vi "Collector.vi"(11 "MechanismMetrics in":T1) -> (3 "MechanismMetrics out":T1)   [LabVIEW 2014]
uses:
  <vilib>/Rock Robotics/WPI/Solenoid/WPI_SolenoidValue.ctl
  Lifter States.ctl
  <vilib>/Rock Robotics/WPI/Solenoid/WPI_SolenoidSetEnum.vi
  MechanismMetrics.ctl
  Auto Lifter States.ctl
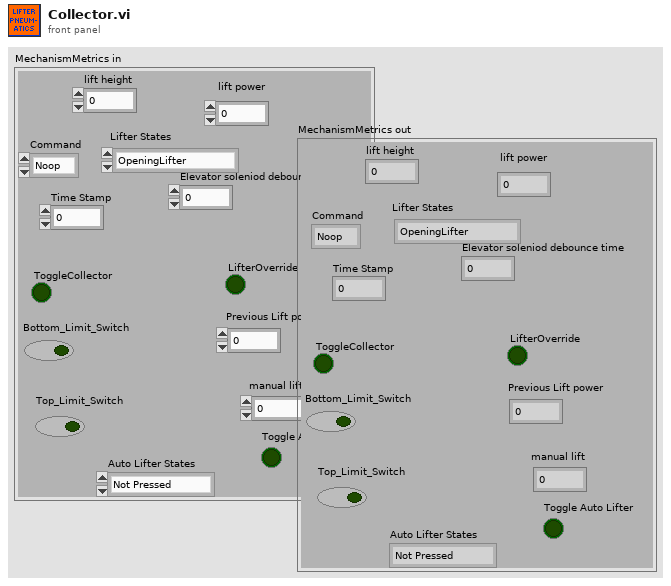
[diagram p1: front panel]
types:
  T1 = typedef "MechanismMetrics.ctl" = cluster{"lift height":dbl, "Command":enum16{"Noop", "Flagged"}, "Time Stamp":u32, "ToggleCollector":bool, "Bottom_Limit_Switch ":bool, "Top_Limit_Switch":bool, "lift power":dbl, "Elevator soleniod debounce time   ":dbl, "LifterOverride":bool, "Previous Lift power":dbl, "manual lift":dbl, "Lifter States":T2, "Auto Lifter States":T3, "Toggle Auto Lifter":bool}
  T2 = typedef "Lifter States.ctl" = enum16{"OpeningLifter", "LifterOpen", "ClosingLifter", "LifterClosed"}
  T3 = typedef "Auto Lifter States.ctl" = enum16{"Not Pressed", "Press Detected", "To Setpoint 1", "To Setpoint 2", "Open Lifter", "Close", "To Setpoint 3"}
  T4 = typedef "WPI_SolenoidValue.ctl" = enum16{"Off", "On", "Forward", "Reverse"}
  T5 = typedef "WPI_SolenoidDevRef.ctl" = cluster{"DevStatus":errorcluster, "Pneumatics Control Module":u8, "Forward Solenoid Channel":T6, "Reverse Solenoid Channel":T6}
  T6 = typedef "WPI_SolenoidChannel.ctl" = enum8{"Solenoid 0", "Solenoid 1", "Solenoid 2", "Solenoid 3", "Solenoid 4", "Solenoid 5", "Solenoid 6", "Solenoid 7", "Invalid"}
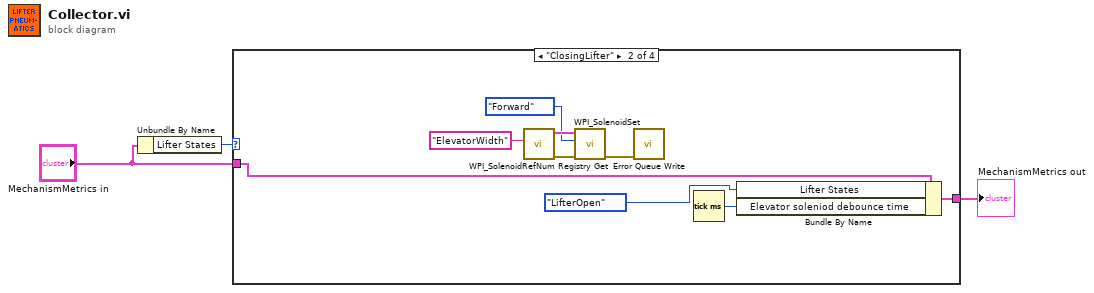
[diagram p0: block diagram]
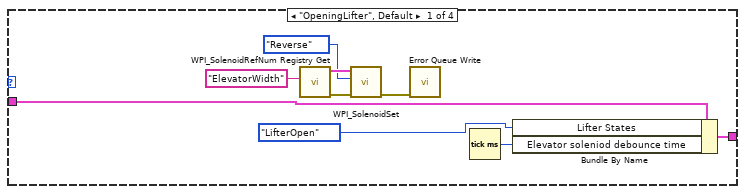
[diagram p2: hidden frame]
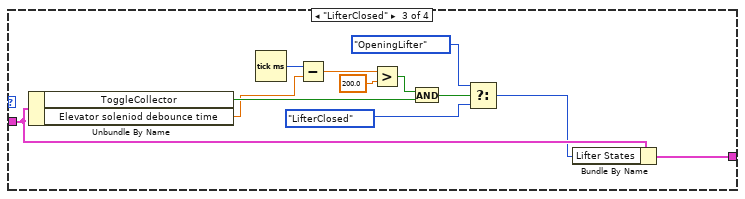
[diagram p3: hidden frame]
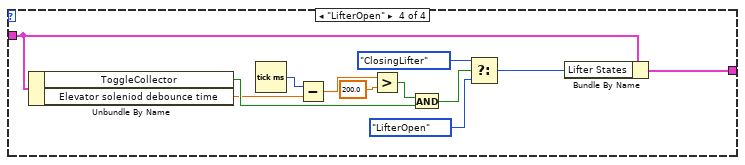
[diagram p4: hidden frame]
diagram:
  n1 = Unbundle By Name("MechanismMetrics in") -> ("Lifter States"=w2:T2)
  n2 = case shown="\"ClosingLifter\"" w2 {
    tunnel: "MechanismMetrics in" -> [w12 w17 w31 w43]
    tunnel: [w7 w16 w30 w44] -> w3
    frame "OpeningLifter", Default {
      n3 = call <vilib>:"WPI_SolenoidRefNum Registry Get.vi"("refnum name"="ElevatorWidth") -> ("error out"=w11:errorcluster, "SolenoidDevRef"=w10:T5)  [unwired: 9 in]
      n4 = call-poly <vilib>:"WPI_SolenoidSet.vi"("error in (no error)"=w11, "Value"=WPI_SolenoidValue."Reverse", "SolenoidDevRef"=w10) -> ("error out"=w8:errorcluster)  [unwired: 7 in, 1 out]
      n5 = call "Error Queue Write.vi"("error in (no error)"=w8) -> ()  [unwired: 11 in]
      n6 = Tick Count (ms)() -> (millisecond timer value=w5:u32)
      n7 = Bundle By Name(cluster=w12, "Lifter States"=Lifter_States."LifterOpen", "Elevator soleniod debounce time"=w5) -> (w7:T1)
    }
    frame "ClosingLifter" {
      n8 = call <vilib>:"WPI_SolenoidRefNum Registry Get.vi"("refnum name"="ElevatorWidth") -> ("error out"=w19:errorcluster, "SolenoidDevRef"=w20:T5)  [unwired: 9 in]
      n9 = call-poly <vilib>:"WPI_SolenoidSet.vi"("error in (no error)"=w19, "Value"=WPI_SolenoidValue."Forward", "SolenoidDevRef"=w20) -> ("error out"=w21:errorcluster)  [unwired: 7 in, 1 out]
      n10 = call "Error Queue Write.vi"("error in (no error)"=w21) -> ()  [unwired: 11 in]
      n11 = Tick Count (ms)() -> (millisecond timer value=w14:u32)
      n12 = Bundle By Name(cluster=w17, "Lifter States"=Lifter_States."LifterOpen", "Elevator soleniod debounce time"=w14) -> (w16:T1)
    }
    frame "LifterClosed" {
      n13 = Unbundle By Name(w31) -> ("ToggleCollector"=w33:bool, "Elevator soleniod debounce time"=w26:dbl)
      n14 = Tick Count (ms)() -> (millisecond timer value=w27:u32)
      n15 = Subtract(x=w27, y=w26) -> (x-y=w25:dbl)
      n16 = Greater?(x=w25, y=200.0) -> (0:w28:bool)
      n17 = And(x=w28, y=w33) -> (x .and. y?=w29:bool)
      n18 = Select(t=Lifter_States."OpeningLifter" ("Collector States"), s=w29, f=Lifter_States."LifterClosed" ("Collector States")) -> (s? t:f=w23:T2)
      n19 = Bundle By Name(cluster=w31, "Lifter States"=w23) -> (w30:T1)
    }
    frame "LifterOpen" {
      n20 = Unbundle By Name(w43) -> ("ToggleCollector"=w45:bool, "Elevator soleniod debounce time"=w38:dbl)
      n21 = Tick Count (ms)() -> (millisecond timer value=w39:u32)
      n22 = Subtract(x=w39, y=w38) -> (x-y=w40:dbl)
      n23 = Greater?(x=w40, y=200.0) -> (0:w41:bool)
      n24 = And(x=w41, y=w45) -> (x .and. y?=w42:bool)
      n25 = Select(t=Lifter_States."ClosingLifter" ("Lifter States"), s=w42, f=Lifter_States."LifterOpen" ("Lifter States")) -> (s? t:f=w36:T2)
      n26 = Bundle By Name(cluster=w43, "Lifter States"=w36) -> (w44:T1)
    }
  }
  "MechanismMetrics out" <- w3
